vi "Populate Event Register_minimal_test.vi"(8 "error in (no error)":errorcluster, 10 "User Events":refnum<user-event>, 11 "Event Registration Refnum":refnum<event-registration>) -> (0 "error out":errorcluster)   [LabVIEW 2013, in "main.lvlib"]
uses:
  main.lvlib
  Components/Dependencies.llb/Exit Event Ref.ctl
  New Design/Controls/Reference AE Control.ctl
  Components/Dependencies.llb/TLB_Dependencies.lvlib
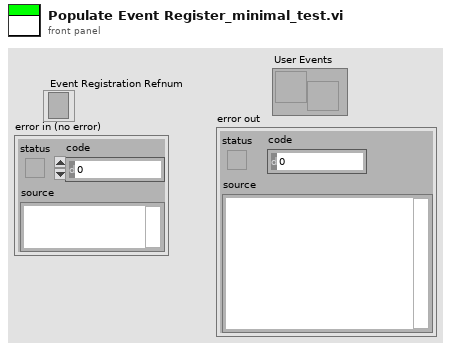
[diagram p1: front panel]
types:
  T1 = typedef "main.lvlib/Reference AE Control.ctl" = enum16{"Initialize", "Set Menu", "Set Profile", "Set Configuration", "Set Configuration_old", "Set Configuration_new", "Set Configuration Method", "Set Acquisition", "Set Data", "Set Journal", "Get"}
  T2 = typedef "main.lvlib/Reference Cluster.ctl" = cluster{"Menu":cluster{"References":cluster{"Stop Acq":refnum<vi>, "MenuExit":refnum<vi>, "MenuStartADC":refnum<vi>, "PersonalInfoString":refnum<vi>, "Profile":refnum<vi>, "Configuration":refnum<vi>, "Acquisition":refnum<vi>, "Data":refnum<vi>, "Journal":refnum<vi>}}, "Profile":cluster{"References":cluster{"Search Patient ID":refnum<vi>, "Name":refnum<vi>, "CommentStr":refnum<vi>, "Listbox Patient ID":refnum<vi>, "ListboxDoctor":refnum<vi>, "ListboxOperator":refnum<vi>, "HospitalName":refnum<vi>, "HospitalDepartment":refnum<vi>, "HospitalAddress":refnum<vi>, "EditHospInfo":refnum<vi>, "Add Patient ID Btn":refnum<vi>, "Query Worklist":refnum<vi>}}, "Configuration":cluster{"References":cluster{"ListboxMeasurementArea":refnum<vi>, "ListboxMeasurementTechnique":refnum<vi>, "ListboxMeasurementMeth":refnum<vi>, "ListboxRightSegmentNr":refnum<vi>, "ListboxLeftSegmentNr":refnum<vi>, "HeightAdjustmentInt":refnum<vi>, "PalpationRight":refnum<vi>, "PalpationLeft":refnum<vi>, "ActivityBox":refnum<vi>}, "New method":cluster{"AddNewMeasurementBtn":refnum<vi>, "Left Time Table":refnum<vi>, "Right Time Table":refnum<vi>}, "Old method":cluster{"LeftArmPressureTable":refnum<vi>, "RightArmPressureTable":refnum<vi>, "SaveArmPressureBtn":refnum<vi>, "Puls":refnum<vi>, "TempTwo":refnum<vi>, "TempOne":refnum<vi>}, "Method":string}, "Acquisition":cluster{"References":cluster{"SegmentAcqString":refnum<vi>, "RingActGraph":refnum<vi>}}, "Data":cluster{"References":cluster{"cmString":refnum<vi>, "AdjustedHeight":refnum<vi>, "Menu":refnum<vi>, "Tangent On/Off":refnum<vi>, "FilterControl":refnum<vi>}}, "Journal":cluster{"References":cluster{"ReportSelection":refnum<vi>, "Data":refnum<vi>, "GenerateReport":refnum<vi>, "Menu":refnum<vi>, "Send To PACS":refnum<vi>}}}
  T3 = cluster{"Stop Acq":refnum<vi>, "MenuExit":refnum<vi>, "MenuStartADC":refnum<vi>, "PersonalInfoString":refnum<vi>, "Profile":refnum<vi>, "Configuration":refnum<vi>, "Acquisition":refnum<vi>, "Data":refnum<vi>, "Journal":refnum<vi>}
  T4 = cluster{"Search Patient ID":refnum<vi>, "Name":refnum<vi>, "CommentStr":refnum<vi>, "Listbox Patient ID":refnum<vi>, "ListboxDoctor":refnum<vi>, "ListboxOperator":refnum<vi>, "HospitalName":refnum<vi>, "HospitalDepartment":refnum<vi>, "HospitalAddress":refnum<vi>, "EditHospInfo":refnum<vi>, "Add Patient ID Btn":refnum<vi>, "Query Worklist":refnum<vi>}
  T5 = cluster{"SegmentAcqString":refnum<vi>, "RingActGraph":refnum<vi>}
  T6 = cluster{"cmString":refnum<vi>, "AdjustedHeight":refnum<vi>, "Menu":refnum<vi>, "Tangent On/Off":refnum<vi>, "FilterControl":refnum<vi>}
  T7 = cluster{"ReportSelection":refnum<vi>, "Data":refnum<vi>, "GenerateReport":refnum<vi>, "Menu":refnum<vi>, "Send To PACS":refnum<vi>}
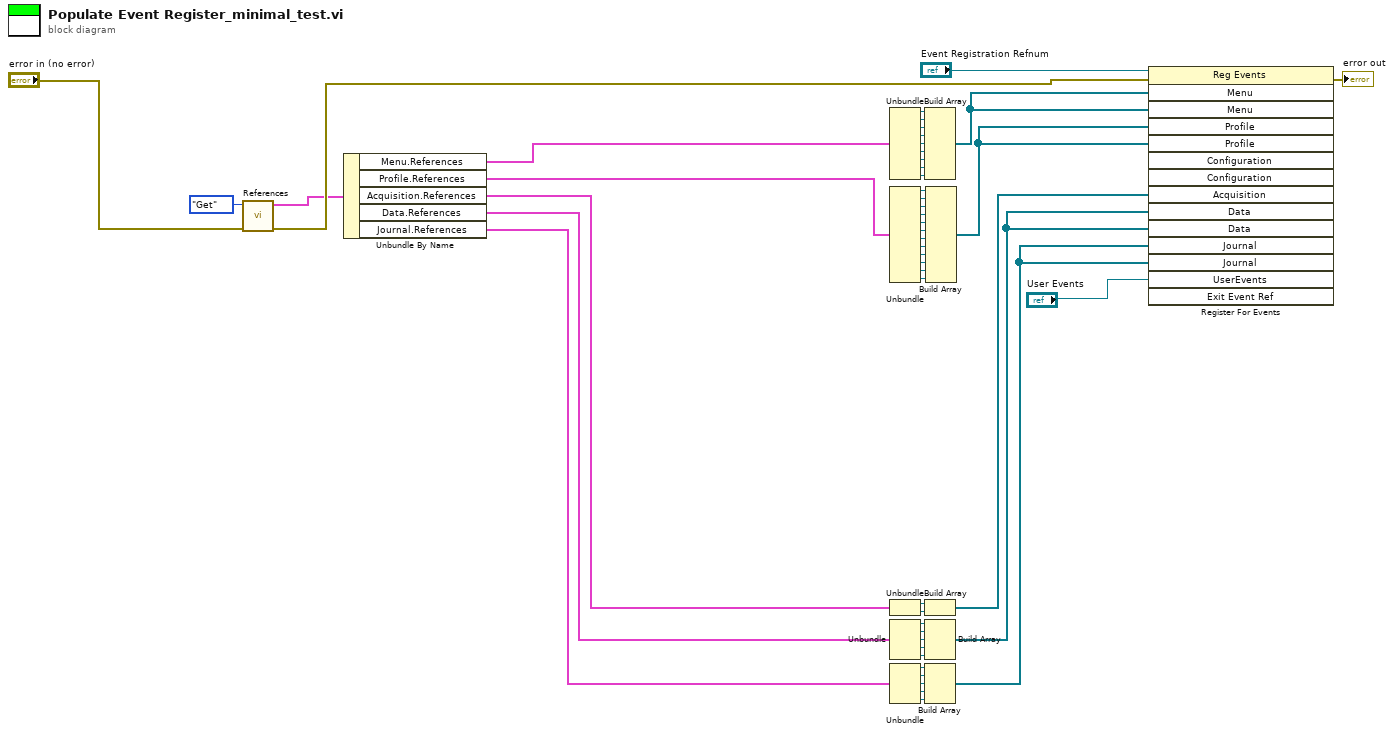
[diagram p0: block diagram]
diagram:
  n1 = call "References.vi"("error in"="error in (no error)", "Reference AE Control"=Reference_AE_Control."Get") -> ("error out"=w4:errorcluster, "Cluster out"=w1:T2)  [unwired: 8 in]
  n2 = Unbundle By Name(w1) -> ("Menu.References"=w48:T3, "Profile.References"=w41:T4, "Acquisition.References"=w28:T5, "Data.References"=w24:T6, "Journal.References"=w17:T7)
  n3 = Unbundle(w48) -> ("Stop Acq"=w47:refnum<vi>, "MenuExit"=w46:refnum<vi>, "MenuStartADC"=w45:refnum<vi>, "PersonalInfoString"=w44:refnum<vi>, "Profile"=w43:refnum<vi>, "Configuration"=w10:refnum<vi>, "Acquisition"=w9:refnum<vi>, "Data"=w8:refnum<vi>, "Journal"=w7:refnum<vi>)
  n4 = Unbundle(w41) -> ("Search Patient ID"=w40:refnum<vi>, "Name"=w39:refnum<vi>, "CommentStr"=w38:refnum<vi>, "Listbox Patient ID"=w37:refnum<vi>, "ListboxDoctor"=w36:refnum<vi>, "ListboxOperator"=w35:refnum<vi>, "HospitalName"=w34:refnum<vi>, "HospitalDepartment"=w33:refnum<vi>, "HospitalAddress"=w32:refnum<vi>, "EditHospInfo"=w31:refnum<vi>, "Add Patient ID Btn"=w30:refnum<vi>, "Query Worklist"=w2:refnum<vi>)
  n5 = Unbundle(w28) -> ("SegmentAcqString"=w27:refnum<vi>, "RingActGraph"=w26:refnum<vi>)
  n6 = Unbundle(w24) -> ("cmString"=w23:refnum<vi>, "AdjustedHeight"=w22:refnum<vi>, "Menu"=w21:refnum<vi>, "Tangent On/Off"=w20:refnum<vi>, "FilterControl"=w19:refnum<vi>)
  n7 = Unbundle(w17) -> ("ReportSelection"=w16:refnum<vi>, "Data"=w15:refnum<vi>, "GenerateReport"=w14:refnum<vi>, "Menu"=w13:refnum<vi>, "Send To PACS"=w3:refnum<vi>)
  n8 = Build Array(w47, w46, w45, w44, w43, w10, w9, w8, w7) -> (w42:refnum<vi>[])
  n9 = Build Array(w27, w26) -> (w25:refnum<vi>[])
  n10 = Build Array(w23, w22, w21, w20, w19) -> (w18:refnum<vi>[])
  n11 = Build Array(w16, w15, w14, w13, w3) -> (w12:refnum<vi>[])
  n12 = Build Array(w40, w39, w38, w37, w36, w35, w34, w33, w32, w31, w30, w2) -> (w29:refnum<vi>[])
  n13 = register-events(reference="Event Registration Refnum", error in=w4, w42, w42, w29, w29, w25, w18, w18, w12, w12, "User Events") -> (error out=→"error out":errorcluster)  [unwired: 3 in, 1 out]
